vi "-8344 Invalid Cell Value Type--error.vi"(8 "error in":errorcluster) -> (0 "error out":errorcluster)   [LabVIEW 2019, in "Open Xml.lvlib"]
uses:
  Open Xml.lvlib
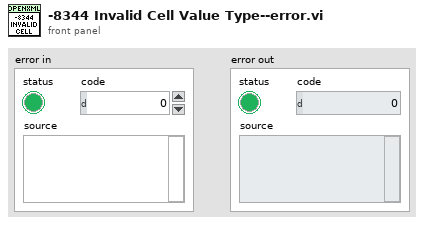
[diagram p1: front panel]
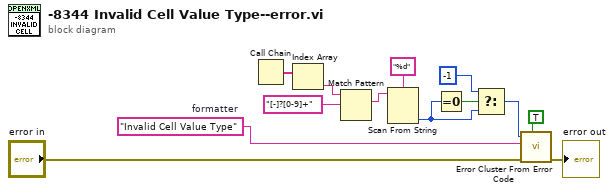
[diagram p0: block diagram]
diagram:
  w11 = "Invalid Cell Value Type"  # formatter
  n1 = Call Chain() -> (call chain=w3:string[])
  n2 = Index Array(array=w3) -> (element=w8:string)  [unwired: 1 in]
  n3 = Match Pattern(string=w8, regular expression="[-]?[0-9]+") -> (match substring=w9:string)  [unwired: 1 in, 3 out]
  n4 = Scan From String(format string="%d", input string=w9) -> (output 1=w5:i32)  [unwired: 3 in, 3 out]
  n5 = Equal To 0?(x=w5) -> (x = 0?=w6:bool)
  n6 = Select(t=-1, s=w6, f=w5) -> (s? t:f=w2:i32)
  n7 = call <vilib>:"Error Cluster From Error Code.vi"("show call chain? (False)"=TRUE, "error in (no error)"="error in", "error message (\"\")"=w11, "error code (0)"=w2) -> ("error out"=→"error out":errorcluster)  [unwired: 5 in]
